vi "JYSlits.vi"(0 "JYMONOLib.IJYMonoReqd In":refnum<k7>, 1 "Slit":u16(ring) items=["Front Entrance", "Side Entrance", "Front Exit", "Side Exit", "First Intermediate", "Second Intermediate"], 2 "UniqueID":string, 3 "error in (no error)":errorcluster, 4 "Slit Width":dbl) -> (5 "JYMONOLib.IJYMonoReqd Out":refnum<k7>, 6 "error out":errorcluster)   [LabVIEW 2012]
doc: "JYSlits.vi\n\nMoves the specified slit to the specified position. Set the front panel switch to local mode (true) to enter the values from the front panel. Set the front panel switch to false (remote mode) to obtain the slit values programmatically. A valid automation refnum or UniqueID must be supplied. If a uniqueId is supplied the VI will generate a new automation refnum. If a valid refnum is supplied, it will be passed through to the output.\n\nInputs\nAutomation Refnum\nUniqueID\nSlit Number\nSlit Width\nInput Error Cluster\n\n\nOutputs\nAutomation Refnum - \nError cluster\n\n\n\n\n\n\n\n\n\n\n\nInputs -\nMonoRefNum In - LabView automation refnum for this mono\nInput Error Cluster -\n\n-----------------------------------------------------\nOutputs -\nMonoRefnum Out - LabView automation refnum for this mono\nOutput Error Cluster"
panel:
  out "IsBusy":bool
  out "UseUniqueID":bool=TRUE
  in  "Input Mode":bool
  # "Front Panel Operation"
  # "Remote Operation"
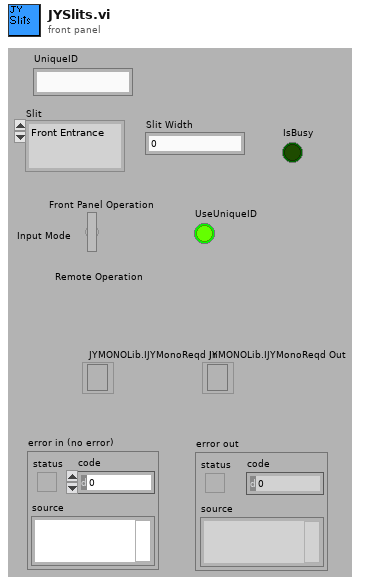
[diagram p1: front panel]
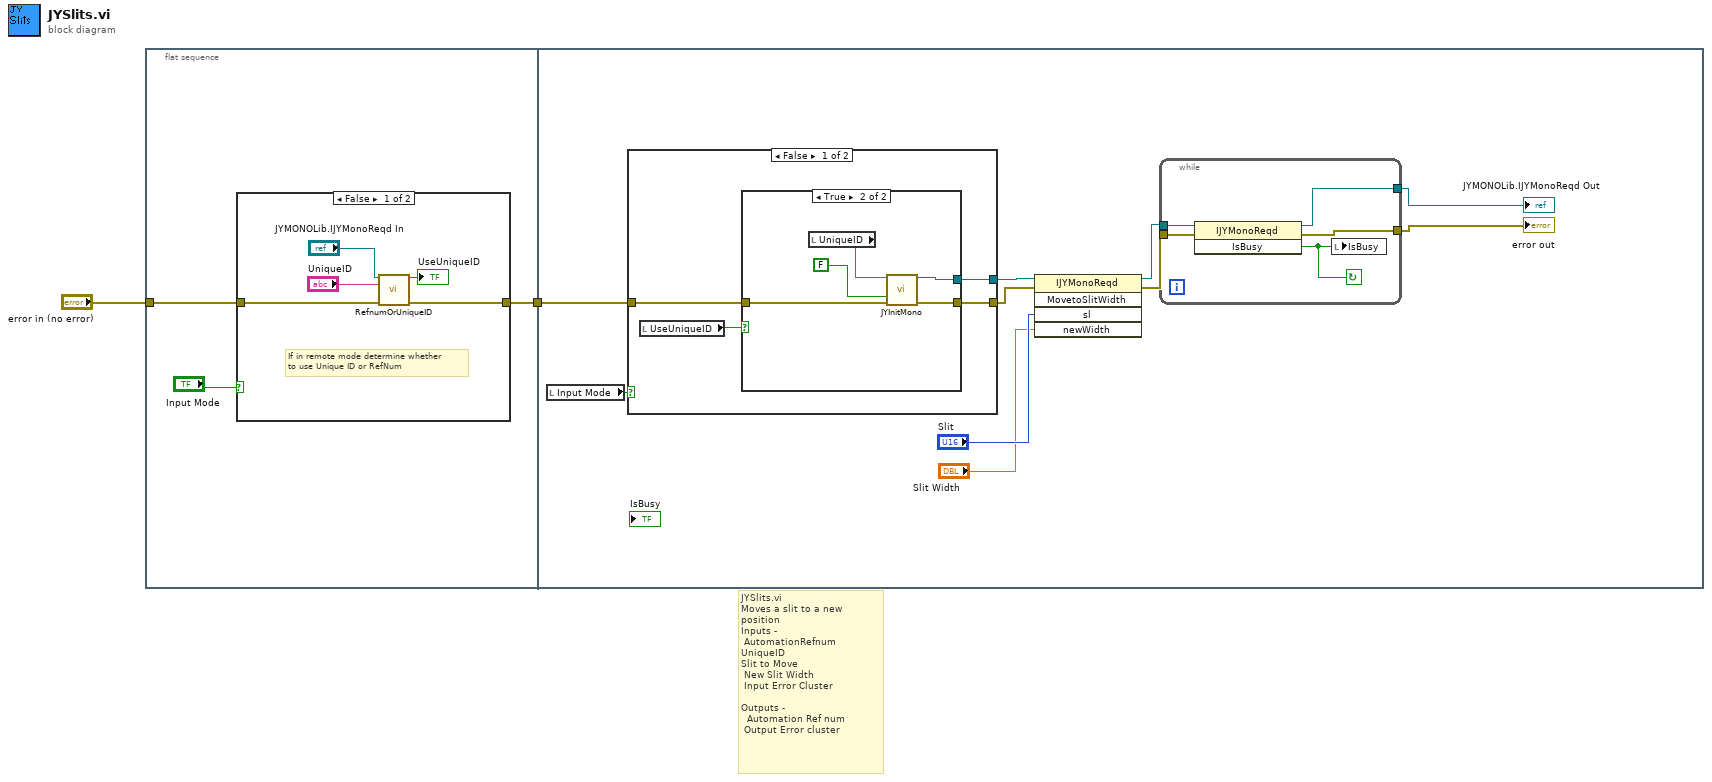
[diagram p0: block diagram]
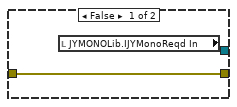
[diagram p3: hidden frame]
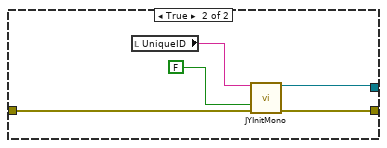
[diagram p4: hidden frame]
diagram:
  # "JYSlits.vi\nMoves a slit to a new position\nInputs - \n AutomationRefnum\nUniqueID\nSlit to Move\n New Slit Width\n Input Error Cluster\n\nOutputs -\n  Automation Ref num\n Output Error cluster"
  n1 = flat-sequence {
    tunnel: "error in (no error)" -> [w4]
    tunnel: [w3] -> w1
    tunnel: w1 -> [w20]
    frame #0 {
      n2 = case shown="False" "Input Mode" {
        tunnel: w4 -> [w10 w11]
        tunnel: [w6 w11] -> w3
        frame False {
          # "If in remote mode determine whether\nto use Unique ID or RefNum"
          n3 = call "RefnumOrUniqueID.vi"("Refnum IN"="JYMONOLib.IJYMonoReqd In", "String in"="UniqueID", "error in (no error)"=w10) -> ("UseUniqueID"=→"UseUniqueID":bool, "error out"=w6:errorcluster)  [unwired: 11 out]
        }
        frame True {
        }
      }
    }
    frame #1 {
      n4 = local read "Input Mode"() -> (w21:bool)
      n5 = case shown="False" w21 {
        tunnel: w20 -> [w29 w40]
        tunnel: [w28 w38] -> w18
        tunnel: [w27 w39] -> w19
        frame False {
          n6 = local read "UseUniqueID"() -> (w30:bool)
          n7 = case shown="True" w30 {
            tunnel: w29 -> [w31 w35]
            tunnel: [w31 w34] -> w28
            tunnel: [w32 w33] -> w27
            frame False {
              n8 = local read "JYMONOLib.IJYMonoReqd In"() -> (w32:refnum<k7>)
            }
            frame True {
              n9 = local read "UniqueID"() -> (w37:string)
              n10 = call "JYInitMono.vi"("Unique ID"=w37, "Force Init"=FALSE, "error in (no error)"=w35) -> ("Mono RefNum out"=w33:refnum<k7>, "error out"=w34:errorcluster)  [unwired: 1 in, 10 out]
            }
          }
        }
        frame True {
          n11 = local read "UniqueID"() -> (w42:string)
          n12 = call "JYInitMono.vi"("Unique ID"=w42, "Force Init"=FALSE ("OK"), "error in (no error)"=w40) -> ("Mono RefNum out"=w39:refnum<k7>, "error out"=w38:errorcluster)  [unwired: 1 in, 10 out]
        }
      }
      n13 = invoke class="IJYMonoReqd" method="MovetoSlitWidth"(reference=w19, error in=w18, "sl"="Slit", "newWidth"="Slit Width") -> (reference out=w17:refnum<k7>, error out=w16:errorcluster)  [unwired: 1 in, 3 out]
      n14 = while {
        tunnel: w17 -> [w25]
        tunnel: w16 -> [w24]
        tunnel: [w23] -> w15
        tunnel: [w22] -> w14
        stop <- w26 continue-if-true
        n15 = invoke class="IJYMonoReqd" method="IsBusy"(reference=w25, error in=w24) -> (reference out=w23:refnum<k7>, error out=w22:errorcluster, "IsBusy"=w26:bool)  [unwired: 1 in]
        n16 = local write "IsBusy"(w26) -> ()
      }
      "error out" <- w14
      "JYMONOLib.IJYMonoReqd Out" <- w15
    }
  }
